vi "Compute IP Header Checksum.vi"(11 "IP Header":u8[](array[numeric]) format="%.0x") -> (3 "Checksum":u8[](array[numeric]))   [LabVIEW 2020, in "EthFrameManagement.lvlib"]
uses:
  EthFrameManagement.lvlib
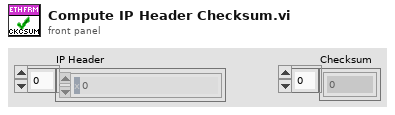
[diagram p1: front panel]
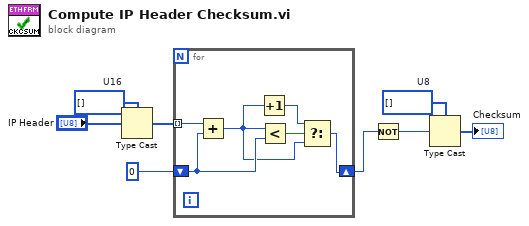
[diagram p0: block diagram]
diagram:
  w2 = u8[] []  # U8
  w8 = u16[] []  # U16
  n1 = Type Cast(type=w8, x="IP Header") -> (*(type *) &x=w6:u16[])
  n2 = for {
    tunnel: w6 -> [w14] mode=indexing
    shift-right: [w9] -> w4
    shift-left: u16 0 ("y") -> [w13]
    n3 = Add(x=w14, y=w13) -> (x+y=w10:u16)
    n4 = Increment(x=w10) -> (x+1=w11:u16)
    n5 = Less?(x=w10, y=w13) -> (x < y?=w12:bool)
    n6 = Select(t=w11, s=w12, f=w10) -> (s? t:f=w9:u16)
  }
  n7 = Not(x=w4) -> (.not. x?=w3:u16)
  n8 = Type Cast(type=w2, x=w3) -> (*(type *) &x=→"Checksum":u8[])
